vi "HW_Gantner_DAQ Status FGV.vi"(7 "Oper":T1, 8 "error in":errorcluster caption="错误输入（无错误）", 11 "DAQ Status in":bool=TRUE) -> (0 "error out":errorcluster caption="错误输出", 3 "DAQ Status out":bool=TRUE)   [LabVIEW 2016]
uses:
  Ctrls/Read and Write Ring.ctl
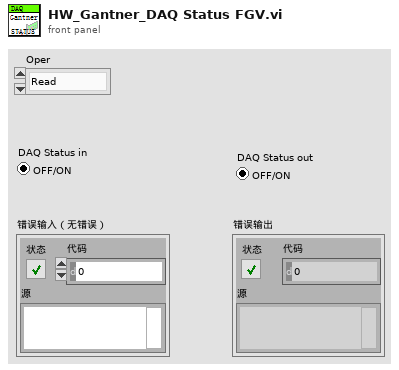
[diagram p1: front panel]
types:
  T1 = typedef "Read and Write Ring.ctl" = enum16{"Read", "Write"}
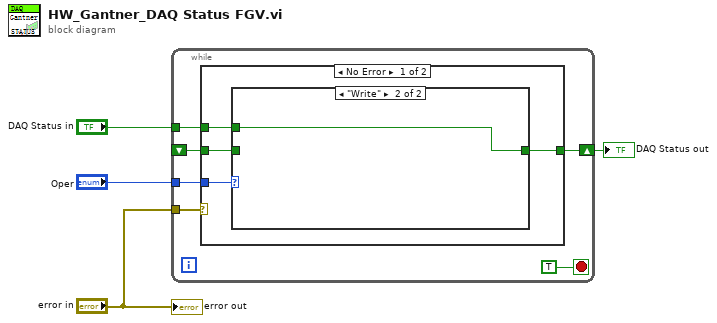
[diagram p0: block diagram]
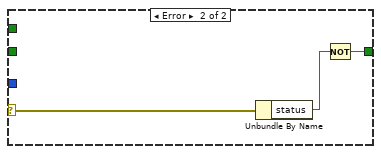
[diagram p3: hidden frame]
diagram:
  n1 = while {
    tunnel: "Oper" -> [w9]
    shift-right: [w7] -> w3
    shift-left: _ -> [w8]
    tunnel: "DAQ Status in" -> [w6]
    tunnel: "error in" -> [w5]
    stop <- TRUE stop-if-true
    n2 = case shown="No Error" w5 {
      selector: w5 -> [_ w19]
      tunnel: w9 -> [w14 _]
      tunnel: w8 -> [w13 _]
      tunnel: [w12 w17] -> w7
      tunnel: w6 -> [w11 _]
      frame No Error {
        n3 = case shown="\"Write\"" w14 {
          tunnel: w13 -> [w15 _]
          tunnel: [w15 w16] -> w12
          tunnel: w11 -> [_ w16]
          frame "Read", Default {
          }
          frame "Write" {
          }
        }
      }
      frame Error {
        n4 = Unbundle By Name(w19) -> ("status"=w18:bool)
        n5 = Not(x=w18) -> (.not. x?=w17:bool)
      }
    }
  }
  "DAQ Status out" <- w3
  "error out" <- "error in"
